vi "MTM2_acceptCommand_applyForces.vi"(8 "error in (no error)":errorcluster, 11 "command_applyForces_Ctl":T1={"private_rcvStamp"=0.0, "axial[72]"=[0.0, 0.0, 0.0, 0.0, 0.0, 0.0, 0.0, 0.0, 0.0, 0.0, 0.0, 0.0, 0.0, 0.0, 0.0, 0.0, 0.0, 0.0, 0.0, 0.0, 0.0, 0.0, 0.0, 0.0, 0.0, 0.0, 0.0, 0.0, 0.0, 0.0, 0.0, 0.0, 0.0, 0.0, 0.0, 0.0, 0.0, 0.0, 0.0, 0.0, 0.0, 0.0, 0.0, 0.0, 0.0, 0.0, 0.0, 0.0, 0.0, 0.0, 0.0, 0.0, 0.0, 0.0, 0.0, 0.0, 0.0, 0.0, 0.0, 0.0, 0.0, 0.0, 0.0, 0.0, 0.0, 0.0, 0.0, 0.0, 0.0, 0.0, 0.0, 0.0], "tangent[6]"=[0.0, 0.0, 0.0, 0.0, 0.0, 0.0]}) -> (0 "error out":errorcluster, 2 "function return":i32, 3 "command_applyForces_Ctl out":T1)   [LabVIEW 2018, in "SALLV_MTM2.lvlib"]
doc: "int MTM2_shm_acceptCommand_applyForcesLV(MTM2_command_applyForcesLV *command_applyForces_Ctl );"
uses:
  DataTypes/command_applyForces.ctl
  SALLV_MTM2.lvlib
  SALLV_MTM2.so
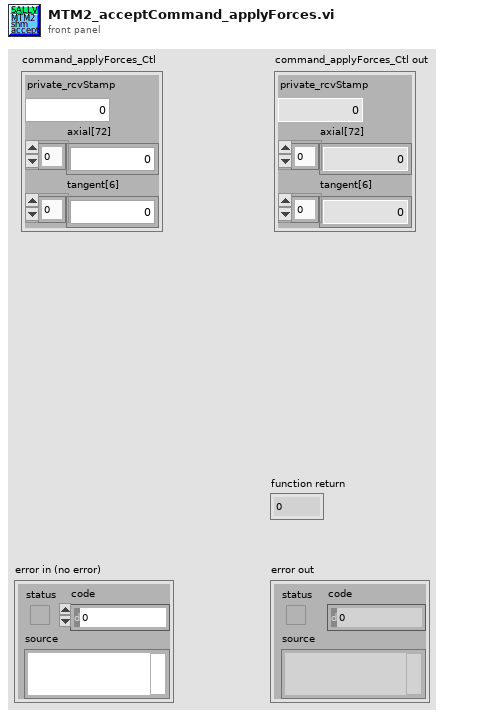
[diagram p1: front panel]
types:
  T1 = typedef "SALLV_MTM2.lvlib/command_applyForces.ctl" = cluster{"private_rcvStamp":dbl, "axial[72]":dbl[], "tangent[6]":dbl[]}
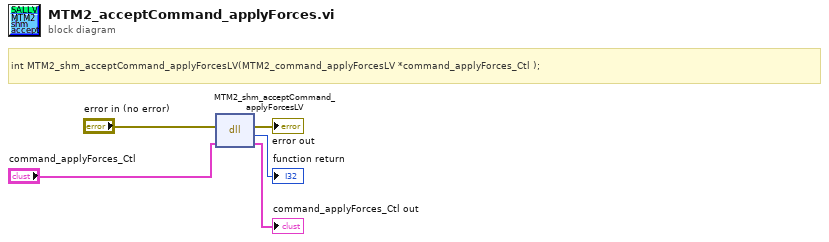
[diagram p0: block diagram]
diagram:
  # "int MTM2_shm_acceptCommand_applyForcesLV(MTM2_command_applyForcesLV *command_applyForces_Ctl );"
  n1 = dll-call lib="home/ttsai/Documents/salTestLabViewApi/SALLV_MTM2/SALLV_MTM2.*" fn="MTM2_shm_acceptCommand_applyForcesLV"(error in="error in (no error)", "command_applyForces_Ctl"="command_applyForces_Ctl") -> (error out=→"error out":errorcluster, →"function return":i32, "command_applyForces_Ctl"=→"command_applyForces_Ctl out":T1)  [unwired: 2 in, 1 out]
